vi "Sub05_01_CoordsVector.vi"(8 "error in (no error)":errorcluster, 11 "appended array":T1(array[cluster])) -> (0 "error out":errorcluster, 3 "String":string)   [LabVIEW 2019]
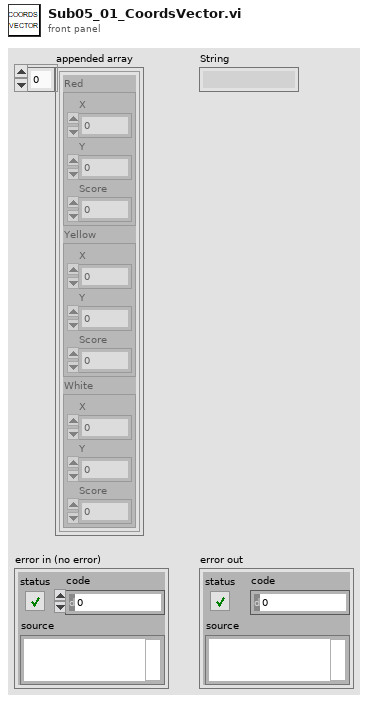
[diagram p1: front panel]
types:
  T1 = cluster{"Red":cluster{"X":u32, "Y":u32, "Score":u32}, "Yellow":cluster{"X":u32, "Y":u32, "Score":u32}, "White":cluster{"X":u32, "Y":u32, "Score":u32}}[]
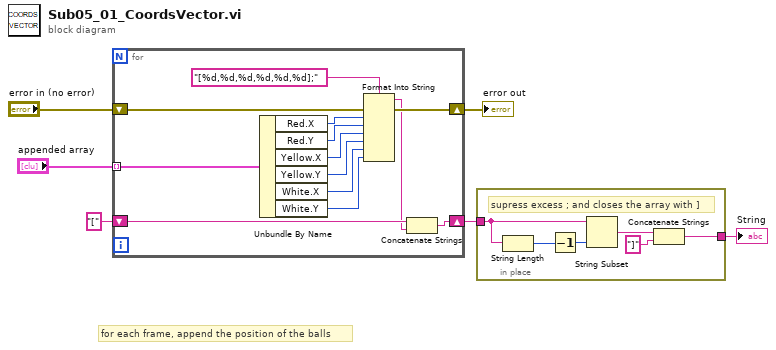
[diagram p0: block diagram]
diagram:
  # "for each frame, append the position of the balls"
  n1 = for {
    tunnel: "appended array" -> [w19] mode=indexing
    shift-right: [w11] -> w2
    shift-left: "[" -> [w12]
    shift-right: [w9] -> w6
    shift-left: "error in (no error)" -> [w10]
    n2 = Unbundle By Name(w19) -> ("Red.X"=w18:u32, "Red.Y"=w17:u32, "Yellow.X"=w16:u32, "Yellow.Y"=w15:u32, "White.X"=w14:u32, "White.Y"=w13:u32)
    n3 = Format Into String(format string="[%d,%d,%d,%d,%d,%d];" ("initial string"), error in=w10, w18, w17, w16, w15, w14, w13) -> (resulting string=w8:string, error out=w9:errorcluster)  [unwired: 1 in]
    n4 = Concatenate Strings(w12, w8) -> (w11:string)
  }
  "error out" <- w6
  n5 = in-place {
    in-place-border: [w25] -> w3
    in-place-border: w2 -> [w22]
    # "supress excess ; and closes the array with ]"
    n6 = String Length(string=w22) -> (length=w20:i32)
    n7 = Decrement(x=w20) -> (x-1=w21:i32)
    n8 = String Subset(string=w22, length (rest)=w21) -> (substring=w23:string)  [unwired: 1 in]
    n9 = Concatenate Strings(w23, "]" ("string")) -> (w25:string)
  }
  "String" <- w3
